vi "Read Roles.vi"(8 "error in (no error)":errorcluster, 11 "GoalKickEnemyPlayVSS in":refnum<class "GoalKickEnemyPlayVSS.lvclass">) -> (0 "error out":errorcluster, 2 "Roles":T1, 3 "GoalKickEnemyPlayVSS out":refnum<class "GoalKickEnemyPlayVSS.lvclass">)   [LabVIEW 2020, in "GoalKickEnemyPlayVSS.lvclass"]
uses:
  GoalKickEnemyPlayVSS.lvclass
  NormalAttackerRoleVSS_class/NormalAttackerRoleVSS.lvclass
  KeeperRoleVSS_class/KeeperRoleVSS.lvclass
  DefenderAreaRoleVSS_class/DefenderAreaRoleVSS.lvclass
  GoalKickEnemyPlayVSS.lvclass/GoalKickEnemyPlayVSS.ctl
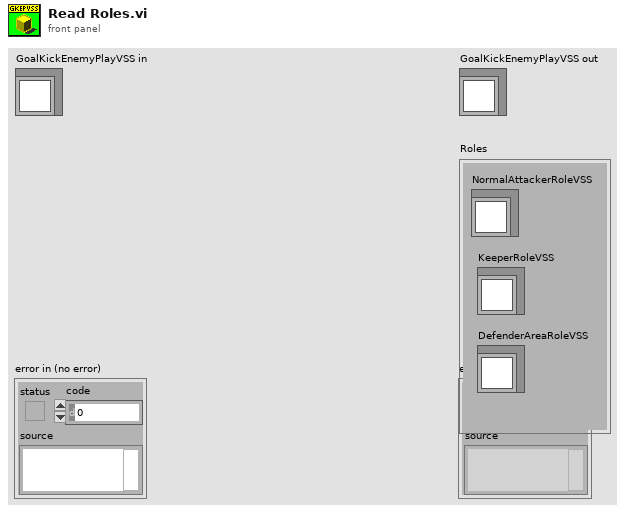
[diagram p1: front panel]
types:
  T1 = cluster{"NormalAttackerRoleVSS":refnum<class "NormalAttackerRoleVSS.lvclass">, "KeeperRoleVSS":refnum<class "KeeperRoleVSS.lvclass">, "DefenderAreaRoleVSS":refnum<class "DefenderAreaRoleVSS.lvclass">}
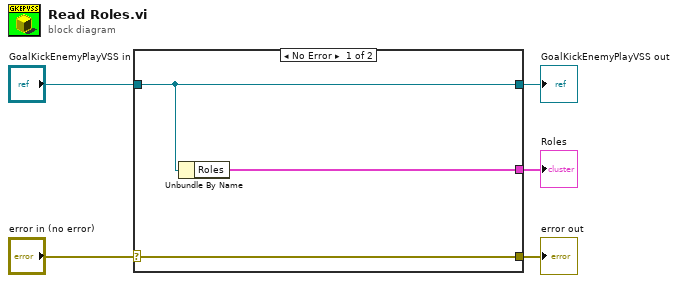
[diagram p0: block diagram]
diagram:
  n1 = case shown="No Error" "error in (no error)" {
    selector: "error in (no error)" -> [w8 w9]
    tunnel: [w8 w9] -> w4
    tunnel: [w7 w10] -> w2
    tunnel: "GoalKickEnemyPlayVSS in" -> [w7 w10]
    tunnel: [w6 _] -> w1
    frame No Error {
      n2 = Unbundle By Name(w7) -> ("Roles"=w6:T1)
    }
    frame Error {
    }
  }
  "error out" <- w4
  "GoalKickEnemyPlayVSS out" <- w2
  "Roles" <- w1
